vi "FPGA Time to LabVIEW Time.vi"(1 "FPGA time (ns)":dbl format="%_28g") -> (0 "LabVIEW time":timestamp)   [LabVIEW 2013, in "FPGA Timekeeper.lvlib"]
doc: "Converts FPGA Time into LabVIEW Time. Note that the FPGA Timekeeper keeps time in nanoseconds starting from January 1st, 1970."
uses:
  FPGA Timekeeper.lvlib
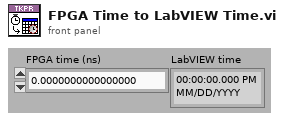
[diagram p1: front panel]
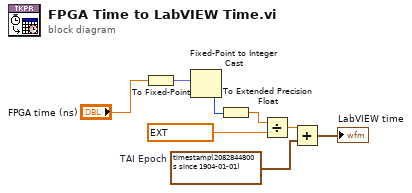
[diagram p0: block diagram]
diagram:
  w6 = timestamp(2082844800 s since 1904-01-01)  # TAI Epoch
  n1 = To Fixed-Point(number="FPGA time (ns)") -> (fixed-point=w2:fxp<+/-,64,44>)  [unwired: 1 in]
  n2 = Fixed-Point to Integer Cast(1:w2) -> (0:w1:i64)
  n3 = To Extended Precision Float(1:w1) -> (0:w4:ext)
  n4 = Divide(x=w4, y=ext 1000000000.0) -> (x/y=w7:ext)
  n5 = Add(x=w7, y=w6) -> (x+y=→"LabVIEW time":timestamp)
